vi "initialise.vi"(8 "error in (no error)":errorcluster, 10 "HWList":string[](array[string]), 11 "BECHWCBasic in":refnum<class "BECHWCBasic.lvclass">) -> (0 "error out":errorcluster, 3 "BECHWCBasic out":refnum<class "BECHWCBasic.lvclass">)   [LabVIEW 2009, in "Hardware.lvlib" / "HWControllers.lvlib" / "BECHWCBasic.lvclass"]
doc: "Initialise the devices in the list"
uses:
  BECHWCBasic.lvclass
  HWController.lvclass
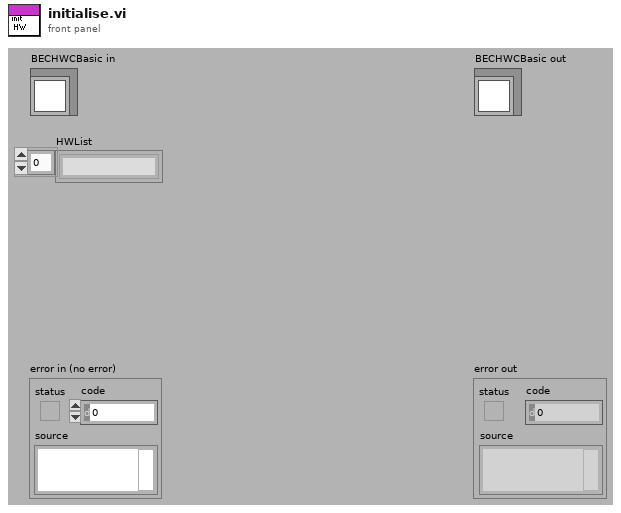
[diagram p1: front panel]
types:
  T1 = enum16{"Ready", "Compiling", "Configured", "Running", "Stopping", "Unresolved Error"}
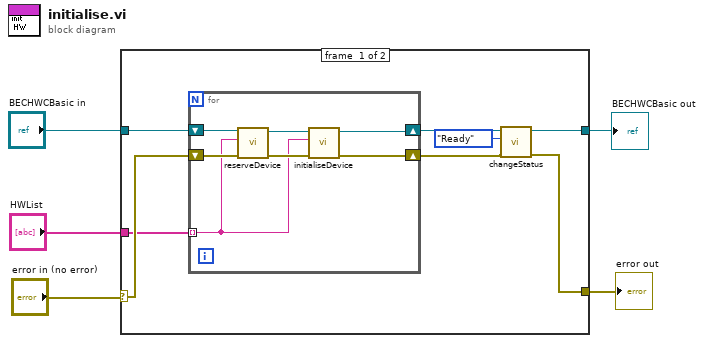
[diagram p0: block diagram]
diagram:
  n1 = case shown="No Error" "error in (no error)" {
    selector: "error in (no error)" -> [w12 w21]
    tunnel: "BECHWCBasic in" -> [w13 w22]
    tunnel: [w10 w22] -> w3
    tunnel: [w8 w21] -> w2
    tunnel: "HWList" -> [w11 _]
    frame #0 {
      n2 = for {
        shift-right: [w15] -> w7
        shift-left: w13 -> [w20]
        tunnel: w11 -> [w16] mode=indexing
        shift-right: [w14] -> w9
        shift-left: w12 -> [w19]
        n3 = call "reserveDevice.vi"("error in (no error)"=w19, "deviceName"=w16, "HWController in"=w20) -> ("error out"=w18:errorcluster, "HWController out"=w17:refnum<class "BECHWCBasic.lvclass">)  [unwired: 7 in]
        n4 = call "initialiseDevice.vi"("error in (no error)"=w18, "deviceName"=w16, "BECHWCBasic in"=w17) -> ("error out"=w14:errorcluster, "BECHWCBasic out"=w15:refnum<class "BECHWCBasic.lvclass">)  [unwired: 7 in]
      }
      n5 = call "changeStatus.vi"("error in (no error)"=w9, "status"=T1."Ready", "HWController in"=w7) -> ("error out"=w8:errorcluster, "HWController out"=w10:refnum<class "BECHWCBasic.lvclass">)  [unwired: 7 in]
    }
    frame #1 {
    }
  }
  "error out" <- w2
  "BECHWCBasic out" <- w3
